vi "ReadXML.vi"(6 "Default Number of Elements":i32, 8 "Reinit":bool, 11 "File Path (.xml)":path) -> (0 "File Open Error":errorcluster, 3 "Data":dbl[](array[numeric]))   [LabVIEW 2019]
doc: "Loads an .xml file as an array of doubles. This is the FRC 4265 standard format for robot-specific calibration data. Set the number of default elements to handle situations in which the .xml file is missing."
uses:
  <vilib>/Utility/xml.llb/Read From XML File(array).vi
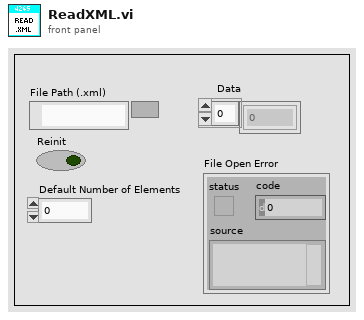
[diagram p1: front panel]
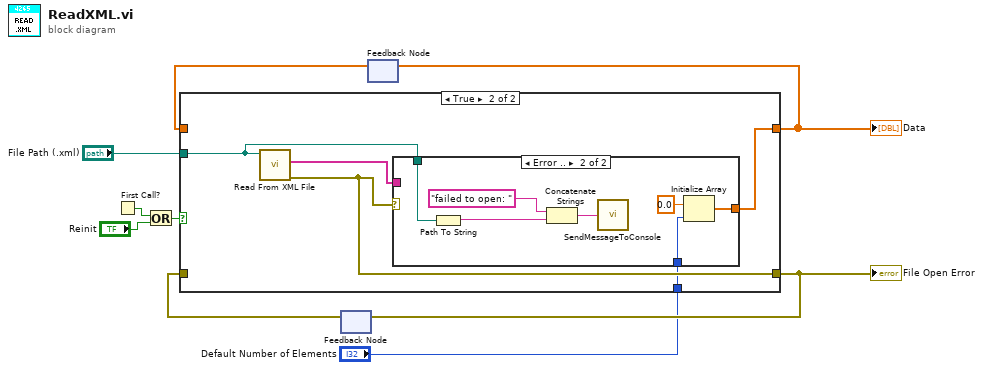
[diagram p0: block diagram]
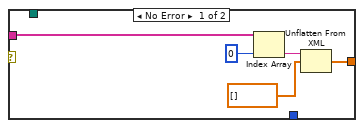
[diagram p3: hidden frame]
diagram:
  n1 = First Call?() -> (First Call?: T/F=w5:bool)
  n2 = Or(x=w5, y="Reinit") -> (x .or. y?=w6:bool)
  n3 = feedback #1() -> (w2:errorcluster)  [unwired: 1 in]
  n4 = feedback #2() -> (w7:dbl[])  [unwired: 1 in]
  n5 = case shown="True" w6 {
    tunnel: "File Path (.xml)" -> [_ w12]
    tunnel: [w11 w15] -> w8
    tunnel: w7 -> [w11 _]
    tunnel: [w10 w14] -> w3
    tunnel: w2 -> [w10 _]
    tunnel: "Default Number of Elements" -> [_ w13]
    frame False {
    }
    frame True {
      n6 = call-poly <vilib>:"Read From XML File.vi"("XML File Path"=w12) -> ("error out"=w14:errorcluster, "XML Elements"=w16:string[])  [unwired: 8 in, 1 out]
      n7 = case shown="Error .." w14 {
        tunnel: w16 -> [w20 _]
        tunnel: [w18 w26] -> w15
        tunnel: w13 -> [_ w27]
        tunnel: w12 -> [_ w22]
        frame No Error {
          n8 = Index Array(array=w20, index=0) -> (element=w19:string)
          n9 = Unflatten From XML(xml string=w19, type=dbl[] [] ("appended array")) -> (value=w18:dbl[])  [unwired: 1 in, 1 out]
        }
        frame Error {
          n10 = Path To String(path=w22) -> (string=w25:string)
          n11 = Concatenate Strings("failed to open: " ("string"), w25) -> (w23:string)
          n12 = call "SendMessageToConsole.vi"("Message String"=w23) -> ()  [unwired: 1 in]
          n13 = Initialize Array(0.0 ("element"), w27) -> (w26:dbl[])
        }
      }
    }
  }
  "Data" <- w8
  "File Open Error" <- w3
  n14 = feedback-in #1(w3) -> ()
  n15 = feedback-in #2(w8) -> ()
